vi "Read.vi"   [LabVIEW 2017, in "Tektronix TDS 200 1000 2000 Series.lvlib"]
doc: "Polymorphic VI that allows users to read one or more waveforms from the oscilloscope ."
uses:
  Tektronix TDS 200 1000 2000 Series.lvlib
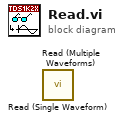
[diagram p0: block diagram]
diagram:
  n1 = call "Read (Single Waveform).vi"() -> ()  [unwired: 9 in, 3 out]
  n2 = call "Read (Multiple Waveforms).vi"() -> ()  [unwired: 9 in, 3 out]
